vi "Construct Build Package Step.vi"(5 "Build Package Step in":refnum<class "Build Package Step.lvclass">, 8 "error in (no error)":errorcluster, 11 "Path":path) -> (0 "error out":errorcluster, 3 "Build Package Step":refnum<class "Build Package Step.lvclass">)   [LabVIEW 2019, in "VIPM.lvlib" / "Build Package Step.lvclass"]
uses:
  Build Package Step.lvclass
  Build Package Step.lvclass/Build Package Step.ctl
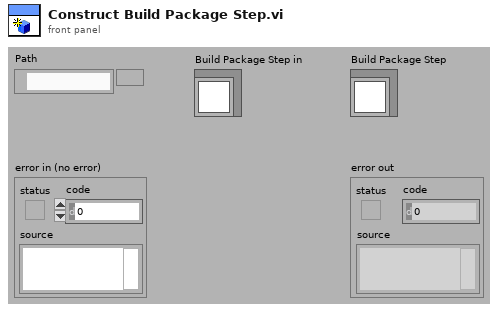
[diagram p1: front panel]
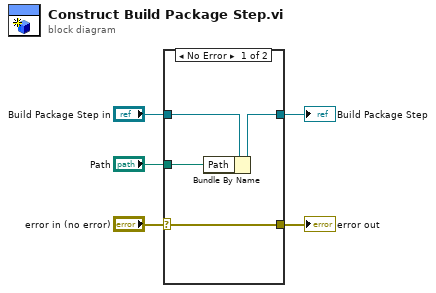
[diagram p0: block diagram]
diagram:
  n1 = case shown="No Error" "error in (no error)" {
    selector: "error in (no error)" -> [w9 w11]
    tunnel: [w9 w11] -> w4
    tunnel: [w7 w10] -> w2
    tunnel: "Build Package Step in" -> [w8 w10]
    tunnel: "Path" -> [w6 _]
    frame No Error {
      n2 = Bundle By Name(cluster=w8, "Path"=w6) -> (w7:refnum<class "Build Package Step.lvclass">)
    }
    frame Error {
    }
  }
  "error out" <- w4
  "Build Package Step" <- w2
